vi "多参数操作日志.vi"(8 "error in (no error)":errorcluster, 11 "data":T1) -> (0 "error out":errorcluster)   [LabVIEW 2016, in "斯坦道原位多参数.lvlib"]
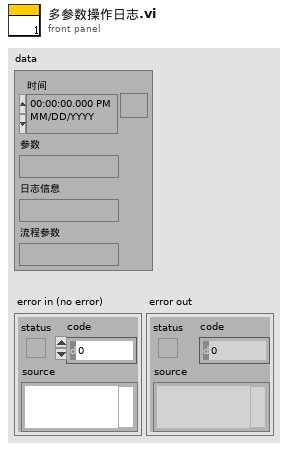
[diagram p1: front panel]
types:
  T1 = typedef "操作日志字段定义.ctl" = cluster{"时间":timestamp, "参数":string, "日志信息":string, "流程参数":string}
  T2 = typedef "数据库类型.ctl" = enum16{"Access", "SQLite"}
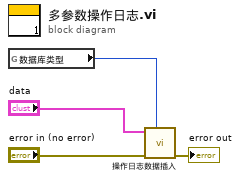
[diagram p0: block diagram]
diagram:
  n1 = global read "多参数断电保存全局变量.vi" "数据库类型"() -> (w2:T2)
  n2 = call "操作日志数据插入.vi"("data"="data", "错误输入（无错误）"="error in (no error)", "数据库类型"=w2) -> ("错误输出"=→"error out":errorcluster)  [unwired: 7 in]
